vi "LV Realterm.vi"() -> ()   [LabVIEW 2009]
uses:
  <vilib>/Instr/_visa.llb/VISA Configure Serial Port (Instr).vi
panel:
  out "Ascii to write hex":string
  in  "SEND":bool
  in  "Ascii to write":string
  out "Incoming Data":string
  in  "stop":bool
  in  "flow control (0:none)":u16(ring) items=["None", "XON/XOFF", "RTS/CTS", "XON/XOFF & RTS/CTS", "DTR/DSR", "XON/XOFF & DTR/DSR"]
  in  "stop bits (10: 1 bit)":u16(ring)=10 items=["1.0"=10, "1.5"=15, "2.0"=20]
  in  "parity (0:none)":enum16{"None", "Odd", "Even", "Mark", "Space"}(ring)
  in  "baud rate (9600)":u32=9600
  in  "data bits (8)":u16=8 min=5 max=8 step=1
  in  "VISA resource name":refnum<visa-resource-name>
  in  "Init":bool
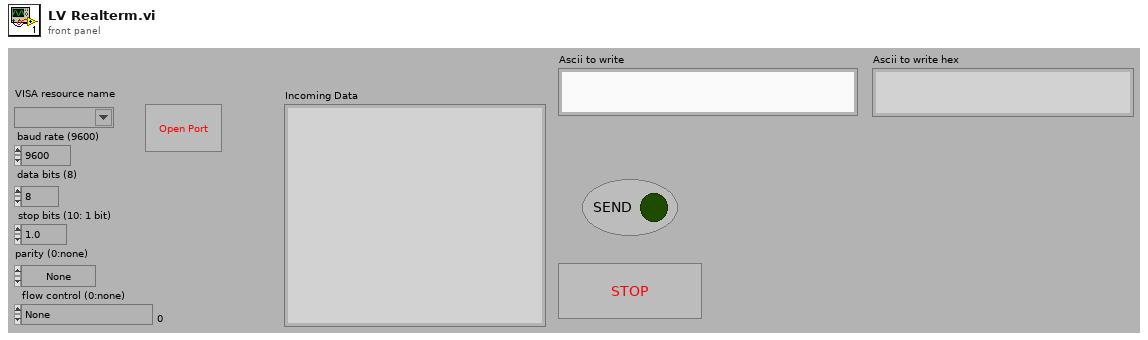
[diagram p1: front panel]
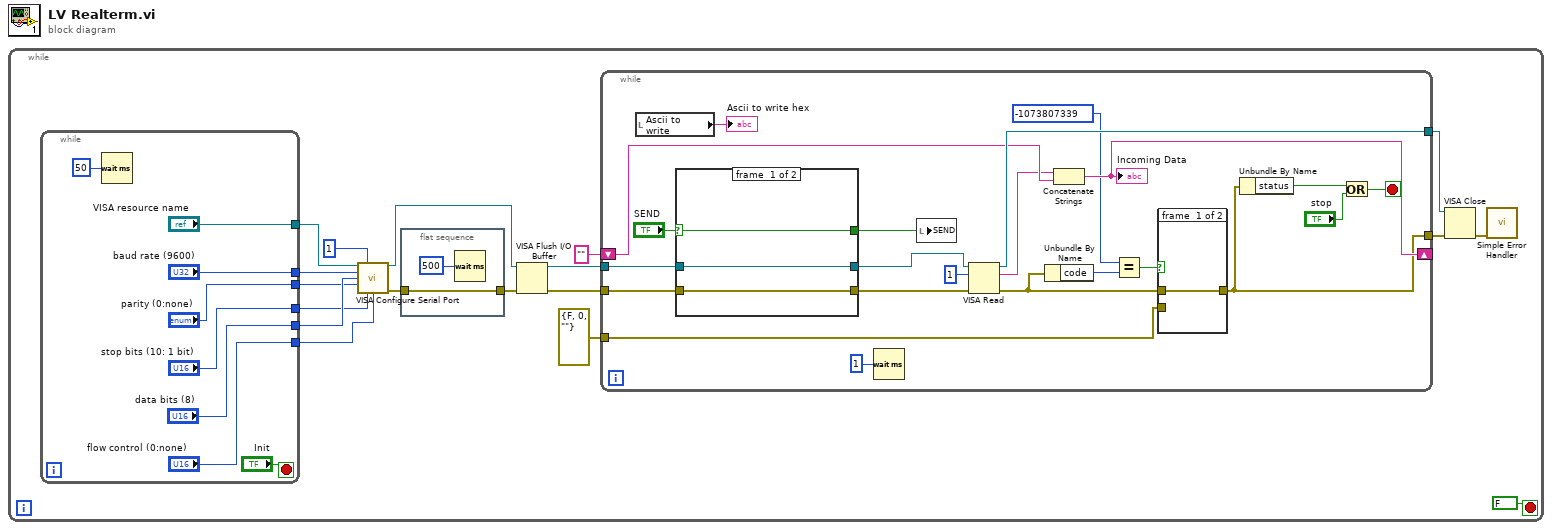
[diagram p0: block diagram]
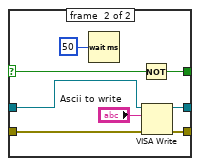
[diagram p3: hidden frame]
diagram:
  n1 = while {
    stop <- FALSE ("stop 2") stop-if-true
    n2 = while {
      tunnel: ["VISA resource name"] -> w18
      tunnel: ["baud rate (9600)"] -> w17
      tunnel: ["data bits (8)"] -> w16
      tunnel: ["parity (0:none)"] -> w15
      tunnel: ["stop bits (10: 1 bit)"] -> w14
      tunnel: ["flow control (0:none)"] -> w13
      stop <- "Init" stop-if-true
      n3 = Wait (ms)(milliseconds to wait=u32 50) -> ()  [unwired: 1 out]
    }
    n4 = call-poly "VISA Configure Serial Port"("VISA resource name"=w18, "timeout (10sec)"=u32 1, "baud rate (9600)"=w17, "data bits (8)"=w16, "parity (0:none)"=w15, "stop bits (10: 1 bit)"=w14, "flow control (0:none)"=w13) -> ("VISA resource name out"=w2:refnum<visa-resource-name>, "error out"=w6:errorcluster)  [unwired: 7 in]
    n5 = flat-sequence {
      tunnel: [w20] -> w5
      tunnel: w6 -> [w20]
      frame #0 {
        n6 = Wait (ms)(milliseconds to wait=u32 500) -> ()  [unwired: 1 out]
      }
    }
    n7 = VISA Flush I/O Buffer(VISA resource name=w2, error in (no error)=w5) -> (VISA resource name out=w3:refnum<visa-resource-name>, error out=w4:errorcluster)  [unwired: 1 in]
    n8 = while {
      tunnel: w3 -> [w35]
      tunnel: w4 -> [w34]
      shift-right: [w39] -> _
      shift-left: "" ("read buffer") -> [w22]
      tunnel: [w25] -> w9
      tunnel: [w38] -> w10
      tunnel: errorcluster {"status"=FALSE, "code"=0, "source"=""} ("error out") -> [w24]
      stop <- w37 stop-if-true
      n9 = local read "Ascii to write"() -> (→"Ascii to write hex":string)
      n10 = case shown="True" "SEND" {
        selector: "SEND" -> [w45 w49]
        tunnel: w35 -> [w47 w55]
        tunnel: w34 -> [w46 w54]
        tunnel: [w47 w53] -> w33
        tunnel: [w46 w52] -> w32
        tunnel: [w45 w50] -> w30
        frame #0 {
        }
        frame #1 {
          n11 = Wait (ms)(milliseconds to wait=u32 50) -> ()  [unwired: 1 out]
          n12 = Not(x=w49) -> (.not. x?=w50:bool)
          n13 = VISA Write(VISA resource name=w55, write buffer="Ascii to write", error in (no error)=w54) -> (VISA resource name out=w53:refnum<visa-resource-name>, error out=w52:errorcluster)  [unwired: 1 out]
        }
      }
      n14 = Wait (ms)(milliseconds to wait=u32 1) -> ()  [unwired: 1 out]
      n15 = local write "SEND"(w30) -> ()
      n16 = VISA Read(VISA resource name=w33, byte count=u32 1, error in (no error)=w32) -> (VISA resource name out=w38:refnum<visa-resource-name>, read buffer=w21:string, error out=w26:errorcluster)  [unwired: 1 out]
      n17 = Unbundle By Name(w26) -> ("code"=w29:i32)
      n18 = Concatenate Strings(w21, w22) -> (w39:string)
      "Incoming Data" <- w39
      n19 = Equal?(x=-1073807339 ("code"), y=w29) -> (x = y?=w27:bool)
      n20 = case shown="True" w27 {
        tunnel: w26 -> [w43 _]
        tunnel: [w43 w44] -> w25
        tunnel: w24 -> [_ w44]
        frame #0 {
        }
        frame #1 {
        }
      }
      n21 = Unbundle By Name(w25) -> ("status"=w36:bool)
      n22 = Or(x=w36, y="stop") -> (x .or. y?=w37:bool)
    }
    n23 = VISA Close(VISA resource name=w10, error in (no error)=w9) -> (error out=w8:errorcluster)
    n24 = call <vilib>:"Simple Error Handler.vi"("error in (no error)"=w8) -> ()  [unwired: 4 in, 5 out]
  }
